vi "Names of plots.vi"(11 "Names of plots":cluster{"Plot.Plot Name":string, i32}[](array[cluster])) -> (3 "Names of plots":cluster{"Plot.Plot Name":string, i32}[](array[cluster]))   [LabVIEW 2020]
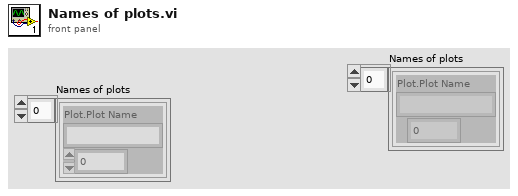
[diagram p1: front panel]
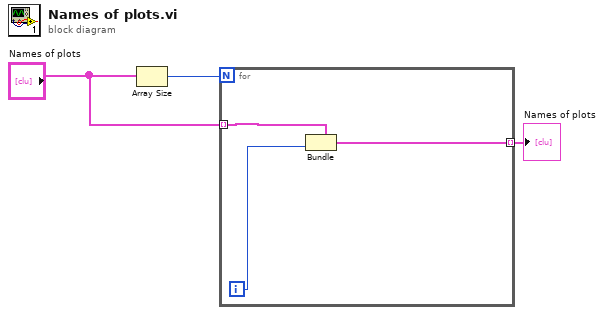
[diagram p0: block diagram]
diagram:
  n1 = Array Size(array="Names of plots") -> (size(s)=w3:i32)
  n2 = for {
    N: w3 -> [_]
    tunnel: "Names of plots" -> [w6] mode=indexing
    tunnel: [w4] -> w1 mode=indexing
    i -> [w5]
    n3 = Bundle(cluster=w6, w5) -> (w4:cluster{"Plot.Plot Name":string, i32})  [unwired: 1 in]
  }
  "Names of plots" <- w1
